vi "Run.vi"(9 "Team in":refnum<class "Team.lvclass">, 11 "MySquare in":refnum<class "MySquare.lvclass">) -> (1 "Team out":refnum<class "Team.lvclass">, 2 "Run Result":T1, 3 "Square out":refnum<class "Square.lvclass">)   [LabVIEW 2020, in "Clones.lvlib" / "MySquare.lvclass"]
doc: "This VI is called on every active square each turn of the game for the square to decide what action to take."
uses:
  MySquare.lvclass
  C:/dev/lv20CE/sol-squarebattle/ProjectTemplates/Source/SummerOfLabVIEW/SquareBattle/template/SquareBattle/Square/Square.lvclass
  SquareBattle/Square/Square.lvclass
  SquareBattle/Run Result.ctl
  SquareBattle/Action.ctl
  SquareBattle/Direction.ctl
  SquareBattle/Team/Team.lvclass
  MySquare.lvclass/MySquare.ctl
  SquareBattle/Square/Square.lvclass/Square.ctl
  SquareBattle/SquareBattle.lvlib
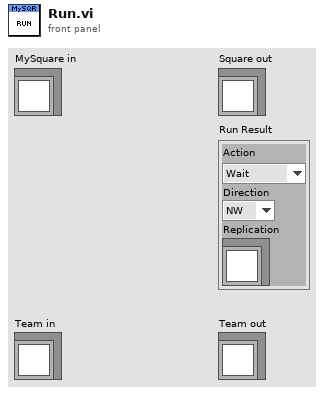
[diagram p1: front panel]
types:
  T1 = typedef "SquareBattle.lvlib/Run Result.ctl" = cluster{"Action":T2, "Direction":T3, "Replication":refnum<class "Square.lvclass">}
  T2 = typedef "SquareBattle.lvlib/Action.ctl" = enum16{"Wait", "Move", "Attack", "Replicate"}
  T3 = typedef "SquareBattle.lvlib/Direction.ctl" = enum16{"NW", "N", "NE", "E", "SE", "S", "SW", "W"}
  T4 = typedef "SquareBattle.lvlib/Location Status.ctl" = cluster{"Empty":bool, "Friend":bool, "Enemy":bool}
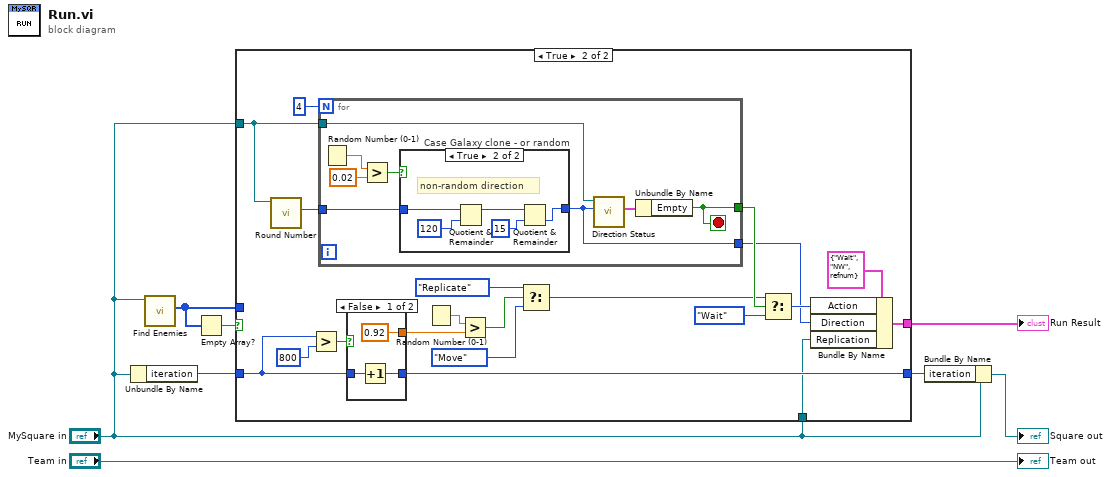
[diagram p0: block diagram]
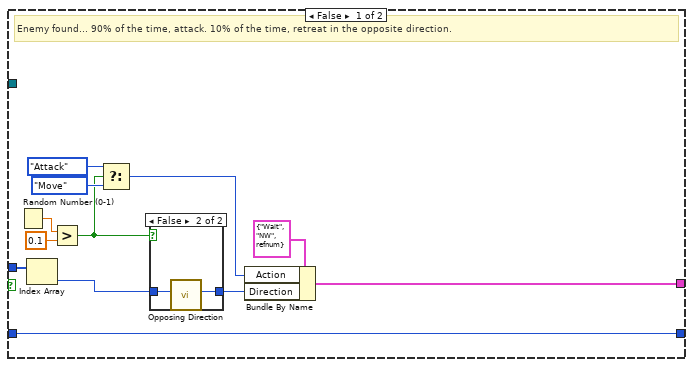
[diagram p2: hidden frame]
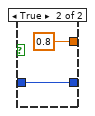
[diagram p4: hidden frame]
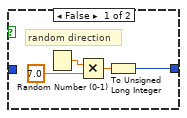
[diagram p5: hidden frame]
diagram:
  n1 = Unbundle By Name("MySquare in") -> ("iteration"=w3:u32)
  n2 = call "Find Enemies.vi"("Square"="MySquare in") -> ("Enemy Directions"=w5:T3[])  [unwired: 10 in]
  n3 = Empty Array?(array=w5) -> (empty?=w6:bool)
  n4 = case shown="True" w6 {
    tunnel: w5 -> [w14 _]
    tunnel: [w20 w40] -> w4
    tunnel: w3 -> [w20 w41]
    tunnel: [w11 w34] -> w2
    tunnel: "MySquare in" -> [_ w37]
    tunnel: "MySquare in" -> [_ w35]
    frame False {
      # "Enemy found... 90% of the time, attack. 10% of the time, retreat in the opposite direction."
      n5 = Random Number (0-1)() -> (number: 0 to 1=w19:dbl)
      n6 = Index Array(array=w14) -> (element=w13:T3)  [unwired: 1 in]
      n7 = Greater?(x=w19, y=0.1) -> (0:w9:bool)
      n8 = Select(t=Action."Attack" ("Action"), s=w9, f=Action."Move" ("Action")) -> (s? t:f=w10:T2)
      n9 = case shown="False" w9 {
        tunnel: w13 -> [w21 w23]
        tunnel: [w21 w22] -> w12
        frame True {
        }
        frame False {
          n10 = call "Opposing Direction.vi"("Direction"=w23) -> ("Opposing Direction"=w22:T3)  [unwired: 10 in]
        }
      }
      n11 = Bundle By Name(cluster=T1 {"Action"=enum."Wait", "Direction"=enum."NW", "Replication"=refnum} ("Run Result"), "Action"=w10, "Direction"=w12) -> (w11:T1)
    }
    frame True {
      n12 = call "Round Number.vi"("Square in"=w37) -> ("Round Number"=w38:u32)  [unwired: 10 in]
      n13 = Greater?(x=w41, y=u32 800) -> (0:w42:bool)
      n14 = for {
        N: 4 -> [_]
        tunnel: w38 -> [w56]
        tunnel: [w49] -> w30
        tunnel: w37 -> [w52]
        tunnel: [w50] -> w33
        stop <- w50 stop-if-true
        n15 = Random Number (0-1)() -> (number: 0 to 1=w54:dbl)
        n16 = Greater?(x=w54, y=0.02) -> (0:w55:bool)
        n17 = case "Case Galaxy clone - or random" shown="True" w55 {
          tunnel: w56 -> [_ w65]
          tunnel: [w57 w64] -> w49
          frame False {
            # "random direction"
            n18 = Random Number (0-1)() -> (number: 0 to 1=w60:dbl)
            n19 = Multiply(x=w60, y=7.0) -> (x*y=w58:dbl)
            n20 = To Unsigned Long Integer(number=w58) -> (unsigned 32bit integer=w57:u32)
          }
          frame True {
            # "non-random direction"
            n21 = Quotient & Remainder(x=w65, y=u32 120) -> (x-y*floor(x/y)=w61:u32)  [unwired: 1 out]
            n22 = Quotient & Remainder(x=w61, y=u32 15) -> (floor(x/y)=w64:u32)  [unwired: 1 out]
          }
        }
        n23 = call "Direction Status.vi"("Direction"=w49, "Square"=w52) -> ("Status"=w51:T4)  [unwired: 8 in, 1 out]
        n24 = Unbundle By Name(w51) -> ("Empty"=w50:bool)
      }
      n25 = case shown="False" w42 {
        tunnel: w41 -> [w46 w48]
        tunnel: [w45 w48] -> w40
        tunnel: [0.92 ("y") 0.8 ("y")] -> w25
        frame False {
          n26 = Increment(x=w46) -> (x+1=w45:u32)
        }
        frame True {
        }
      }
      n27 = Random Number (0-1)() -> (number: 0 to 1=w26:dbl)
      n28 = Greater?(x=w26, y=w25) -> (0:w27:bool)
      n29 = Select(t=Action."Replicate" ("Action"), s=w27, f=Action."Move" ("Action")) -> (s? t:f=w24:T2)
      n30 = Select(t=w24, s=w33, f=Action."Wait" ("Action")) -> (s? t:f=w31:T2)
      n31 = Bundle By Name(cluster=T1 {"Action"=enum."Wait", "Direction"=enum."NW", "Replication"=refnum} ("Run Result"), "Action"=w31, "Direction"=w30, "Replication"=w35) -> (w34:T1)
    }
  }
  "Run Result" <- w2
  n32 = Bundle By Name(cluster="MySquare in", "iteration"=w4) -> (→"Square out":refnum<class "MySquare.lvclass">)
  "Team out" <- "Team in"
